vi "hpanel_DO_stream_TTTR.vi"(0 "hydraharp_panel in":refnum<class "hydraharp_panel.lvclass">, 1 "acq_time":i32, 3 "Record Type":T1, 5 "fifo_stream_path":path, 7 "action_for_records":T5, 9 "Stream Notes":string, 11 "error in (no error)":errorcluster, 12 "stop_fifo_event":refnum<event-registration>, 14 "Correlation_settings":T2 {"Lag Settings"."time_start" items=["1 ps"=1, "10 ps"=10, "100 ps"=100, "1 ns"=1000, "10 ns"=10000, "100 ns"=100000, "1 us"=1000000, "10 us"=10000000, "100 us"=100000000, "1 ms"=1000000000, "10 ms"=10000000000, "100 ms"=100000000000, "1 s"=1000000000000, "10 s"=10000000000000, "100 s"=100000000000000]; "Lag Settings"."time_end" items=["1 ps"=1, "10 ps"=10, "100 ps"=100, "1 ns"=1000, "10 ns"=10000, "100 ns"=100000, "1 us"=1000000, "10 us"=10000000, "100 us"=100000000, "1 ms"=1000000000, "10 ms"=10000000000, "100 ms"=100000000000, "1 s"=1000000000000, "10 s"=10000000000000, "100 s"=100000000000000]}) -> (4 "hydraharp_panel out":refnum<class "hydraharp_panel.lvclass">, 15 "error out":errorcluster)   [LabVIEW 2015, in "hydraharp_panel.lvclass"]
uses:
  hydraharp_panel.lvclass
  hydraharp/hydraharp_action_on_records.ctl
  hpanel_correlation_settings.ctl
  hydraharp/hydraharp_correlation_lag_settings.ctl
  hydraharp/hydraharp_time_decades.ctl
  record_type.ctl
  hydraharp/hydraharp.lvclass
  hpanel_messages_to_panel_from_actor_loop.ctl
  hydraharp/hydraharp.lvclass/hydraharp.ctl
  Picoquant_generic/processing_tasks_tdef.ctl
  Picoquant_generic/picoquant_generic.lvclass/picoquant_generic.ctl
  UI/panel_class/panel.lvclass
  Picoquant_generic/picoquant_generic.lvclass
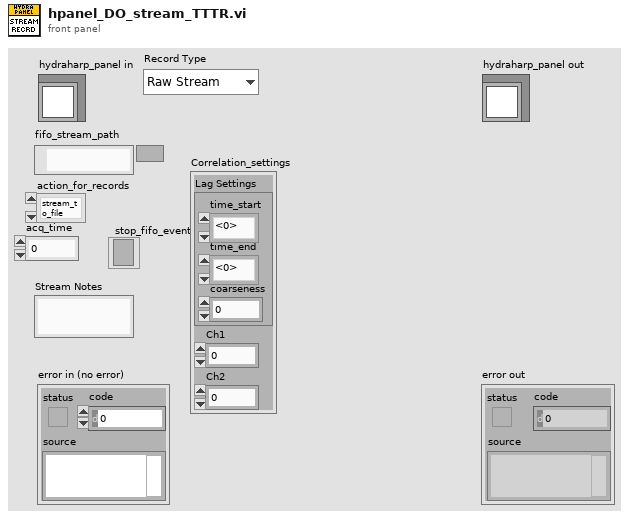
[diagram p1: front panel]
types:
  T1 = typedef "record_type.ctl" = enum16{"Raw Stream", "Processed Records (hdf5)"}
  T2 = typedef "hpanel_correlation_settings.ctl" = cluster{"Lag Settings":T3, "Ch1":u8, "Ch2":u8}
  T3 = typedef "hydraharp_correlation_lag_settings.ctl" = cluster{"time_start":T4, "time_end":T4, "coarseness":i64}
  T4 = typedef "hydraharp_time_decades.ctl" = i64
  T5 = typedef "hydraharp_action_on_records.ctl" = enum16{"stream_to_file", "correlate", "stream to file and correlate", "histogram"}
  T6 = typedef "hpanel_messages_to_panel_from_actor_loop.ctl" = enum16{"reenable_tasks"}
  T7 = typedef "processing_tasks_tdef.ctl" = enum16{"none", "correlate", "histogram"}
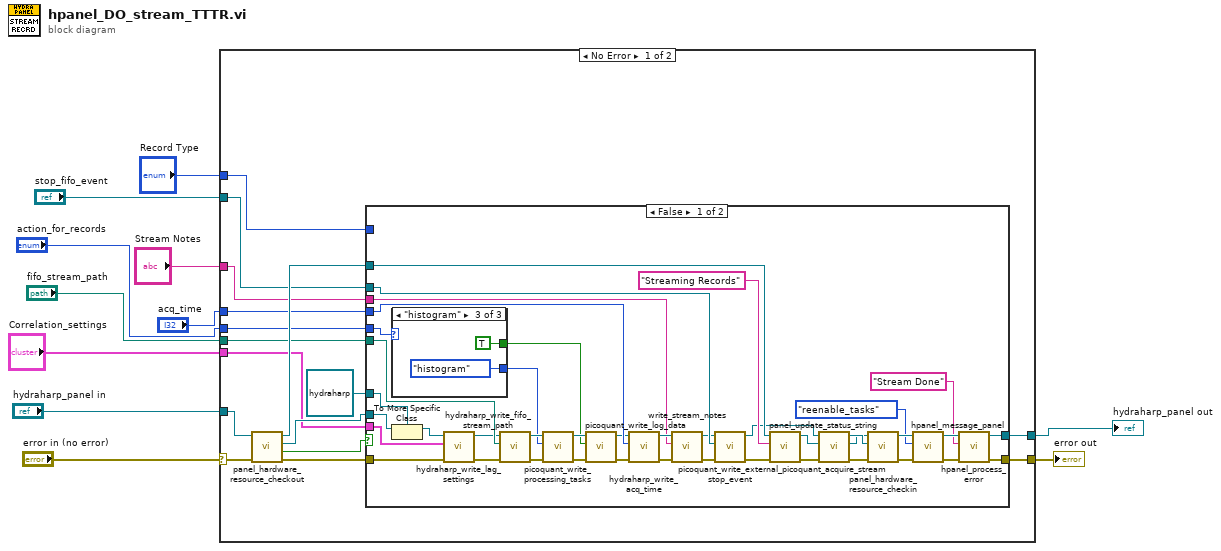
[diagram p0: block diagram]
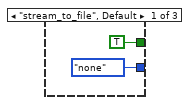
[diagram p2: hidden frame]
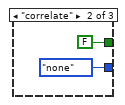
[diagram p3: hidden frame]
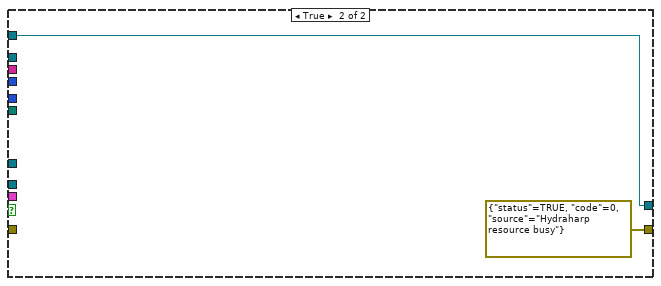
[diagram p4: hidden frame]
diagram:
  n1 = case shown="No Error" "error in (no error)" {
    selector: "error in (no error)" -> [w26 w78]
    tunnel: [w17 w78] -> w10
    tunnel: [w18 w77] -> w8
    tunnel: "hydraharp_panel in" -> [w27 w77]
    tunnel: "fifo_stream_path" -> [w20 _]
    tunnel: "action_for_records" -> [w19 _]
    tunnel: "acq_time" -> [w16 _]
    tunnel: "stop_fifo_event" -> [w15 _]
    tunnel: "Correlation_settings" -> [w14 _]
    tunnel: "Record Type" -> [w13 _]
    tunnel: "Stream Notes" -> [w12 _]
    frame No Error {
      n2 = call "panel_hardware_resource_checkout.vi"("error in (no error)"=w26, "panel in"=w27) -> ("error out"=w22:errorcluster, "timed out?"=w23:bool, "hardware.lvclass"=w25:refnum<class "hardware.lvclass">, "panel out"=w21:refnum<class "hydraharp_panel.lvclass">)  [unwired: 6 in]
      n3 = case shown="False" w23 {
        tunnel: w25 -> [w67 _]
        tunnel: refnum<class "hydraharp.lvclass"> refnum ("hydraharp.lvclass") -> [w68 _]
        tunnel: w22 -> [w59 _]
        tunnel: w21 -> [w65 w75]
        tunnel: w20 -> [w66 _]
        tunnel: w19 -> [w30 _]
        tunnel: [w51 w75] -> w18
        tunnel: [w50 errorcluster {"status"=TRUE, "code"=0, "source"="Hydraharp resource busy"} ("error out")] -> w17
        tunnel: w16 -> [w63 _]
        tunnel: w15 -> [w39 _]
        tunnel: w14 -> [w55 _]
        tunnel: w13 -> [_ _]
        tunnel: w12 -> [w47 _]
        frame False {
          n4 = case shown="\"histogram\"" w30 {
            tunnel: [TRUE FALSE TRUE] -> w29
            tunnel: [processing_tasks_tdef."none" ("processing tasks") processing_tasks_tdef."none" ("processing tasks") processing_tasks_tdef."histogram" ("processing tasks")] -> w28
            frame "stream_to_file", Default {
            }
            frame "correlate" {
            }
            frame "histogram" {
            }
          }
          n5 = To More Specific Class(target class=w68, reference=w67) -> (specific class reference=w57:refnum<class "hydraharp.lvclass">)  [unwired: 1 in, 1 out]
          n6 = call "hydraharp_write_lag_settings.vi"("error in (no error)"=w59, "lag_settings"=w55, "hydraharp in"=w57) -> ("error out"=w58:errorcluster, "hydraharp out"=w56:refnum<class "hydraharp.lvclass">)  [unwired: 7 in]
          n7 = call "hydraharp_write_fifo_stream_path.vi"("error in (no error)"=w58, "fifo_stream_path"=w66, "hydraharp in"=w56) -> ("error out"=w36:errorcluster, "hydraharp out"=w35:refnum<class "hydraharp.lvclass">)  [unwired: 7 in]
          n8 = call "picoquant_write_processing_tasks.vi"("error in (no error)"=w36, "processing tasks"=w28, "picoquant_generic in"=w35) -> ("error out"=w32:errorcluster, "picoquant_generic out"=w34:refnum<class "hydraharp.lvclass">)  [unwired: 7 in]
          n9 = call "picoquant_write_log_data.vi"("error in (no error)"=w32, "log data?"=w29, "picoquant_generic in"=w34) -> ("error out"=w31:errorcluster, "picoquant_generic out"=w33:refnum<class "hydraharp.lvclass">)  [unwired: 7 in]
          n10 = call "hydraharp_write_acq_time.vi"("error in (no error)"=w31, "acq_time"=w63, "hydraharp in"=w33) -> ("error out"=w48:errorcluster, "hydraharp out"=w49:refnum<class "hydraharp.lvclass">)  [unwired: 7 in]
          n11 = call "write_stream_notes.vi"("error in (no error)"=w48, "Stream Notes"=w47, "hydraharp in"=w49) -> ("error out"=w41:errorcluster, "hydraharp out"=w38:refnum<class "hydraharp.lvclass">)  [unwired: 7 in]
          n12 = call "picoquant_write_external_stop_event.vi"("error in (no error)"=w41, "external_stop_event"=w39, "picoquant_generic in"=w38) -> ("error out"=w37:errorcluster, "picoquant_generic out"=w40:refnum<class "hydraharp.lvclass">)  [unwired: 7 in]
          n13 = call-dynamic "panel_update_status_string.vi"("error in (no error)"=w37, "String"="Streaming Records", "hydraharp_panel in"=w65) -> ("error out"=w46:errorcluster, "hydraharp_panel out"=w44:refnum<class "hydraharp_panel.lvclass">)  [unwired: 7 in]
          n14 = call "picoquant_acquire_stream.vi"("error in (no error)"=w46, "picoquant_panel"=w44, "picoquant_generic in"=w40) -> ("error out"=w45:errorcluster, "panel out"=w42:refnum<class "hydraharp_panel.lvclass">, "picoquant_generic out"=w43:refnum<class "hydraharp.lvclass">)  [unwired: 6 in]
          n15 = call "panel_hardware_resource_checkin.vi"("error in (no error)"=w45, "hardware.lvclass"=w43, "panel in"=w42) -> ("error out"=w62:errorcluster, "panel out"=w61:refnum<class "hydraharp_panel.lvclass">)  [unwired: 7 in]
          n16 = call "hpanel_message_panel.vi"("error in (no error)"=w62, "event data"=hpanel_messages_to_panel_from_actor_loop."reenable_tasks", "hydraharp_panel in"=w61) -> ("error out"=w54:errorcluster, "hydraharp_panel out"=w53:refnum<class "hydraharp_panel.lvclass">)  [unwired: 7 in]
          n17 = call "hpanel_process_error.vi"("error in (no error)"=w54, "No Error Message"="Stream Done", "hydraharp_panel in"=w53) -> ("error out"=w50:errorcluster, "hydraharp_panel out"=w51:refnum<class "hydraharp_panel.lvclass">)  [unwired: 7 in]
        }
        frame True {
        }
      }
    }
    frame Error {
    }
  }
  "error out" <- w10
  "hydraharp_panel out" <- w8
